vi "sub_joystick-data-conv.vi"(11 "joystick info-in":T1) -> (2 "cmd":u32, 3 "opval":cluster{dbl, dbl} {"?" format="%-1.1f"; "?" format="%-1.1f"})   [LabVIEW 2021]
uses:
  Ctrl/cmd_common.ctl
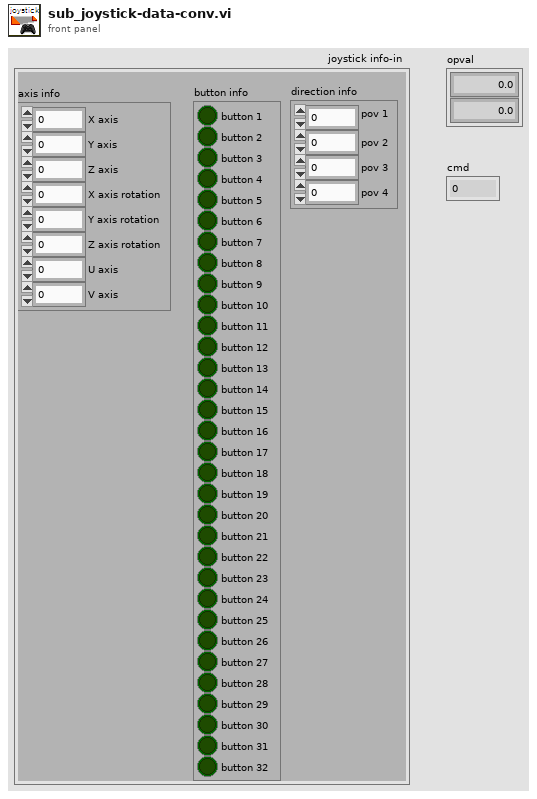
[diagram p1: front panel]
types:
  T1 = cluster{"axis info":cluster{"X axis":i32, "Y axis":i32, "Z axis":i32, "X axis rotation":i32, "Y axis rotation":i32, "Z axis rotation":i32, "U axis":i32, "V axis":i32}, "button info":cluster{"button 1":bool, "button 2":bool, "button 3":bool, "button 4":bool, "button 5":bool, "button 6":bool, "button 7":bool, "button 8":bool, "button 9":bool, "button 10":bool, "button 11":bool, "button 12":bool, "button 13":bool, "button 14":bool, "button 15":bool, "button 16":bool, "button 17":bool, "button 18":bool, "button 19":bool, "button 20":bool, "button 21":bool, "button 22":bool, "button 23":bool, "button 24":bool, "button 25":bool, "button 26":bool, "button 27":bool, "button 28":bool, "button 29":bool, "button 30":bool, "button 31":bool, "button 32":bool}, "direction info":cluster{"pov 1":i32, "pov 2":i32, "pov 3":i32, "pov 4":i32}}
  T2 = typedef "system_hw.ctl" = cluster{"UGV":enum16{"none", "Scout", "RLCar", "ASV", "Bunker"}, "Lidar 1":enum16{"none", "VLP16", "TIM571", "RPLidar A2", "RPLidar A3", "Ouster"}, "Lidar 2":enum16{"none", "VLP16", "TIM571", "RPLidar A2", "RPLidar A3"}, "GPS":enum16{"none", "NMEA 232", "Custom", "tbd"}, "Camera 1":enum16{"none", "C920", "C922", "GT1290C", "MS LifeCam"}, "Joystick":enum16{"none", "joystick"}, "sound":enum16{"none", "speaker"}, "IMU":enum16{"none", "MW-AHRSv1", "VN-100", "MTi-630", "Ellipse-D", "WT901CTTL"}, "Led":enum16{"none", "LedMatrix 8x32"}, "Camera 2":enum16{"none", "C920", "C922", "GT1290C", "MS LifeCam"}, "Camera 3":enum16{"none", "C920", "C922", "GT1290C", "MS LifeCam"}, "Camera 4":enum16{"none", "C920", "C922", "GT1290C", "MS LifeCam"}}
  T3 = enum16{"none", "Scout", "RLCar", "ASV", "Bunker"}
  T4 = typedef "cmd_common.ctl" = enum16{"read", "write"}
  T5 = typedef "joystick cfg.ctl" = cluster{"steer limit":cluster{"scale":dbl, "offset":dbl}, "speed limit":cluster{"min":dbl, "max":dbl}, "Axis":cluster{"man":dbl, "auto":dbl, "angular":T6, "linear":T6, "linear inv":bool, "ang inv":bool}}
  T6 = typedef "joy-axis.ctl" = enum16{"X axis", "Y axis", "Z axis", "X rotation", "Y rotation", "Z rotation", "U axis", "V axis"}
  T7 = cluster{"X axis":i32, "Y axis":i32, "Z axis":i32, "X axis rotation":i32, "Y axis rotation":i32, "Z axis rotation":i32, "U axis":i32, "V axis":i32}
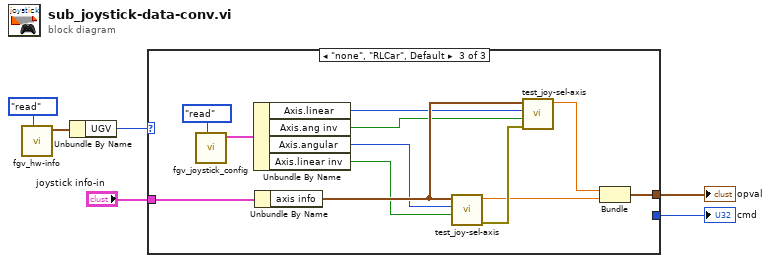
[diagram p0: block diagram]
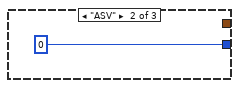
[diagram p3: hidden frame]
diagram:
  n1 = call "fgv_hw-info.vi"("cmd"=enum16{"write", "read"}."read") -> ("HW info out"=w1:T2)  [unwired: 10 in]
  n2 = Unbundle By Name(w1) -> ("UGV"=w3:T3)
  n3 = case shown="\"none\", \"RLCar\", Default" w3 {
    tunnel: [_ _ w10] -> w6
    tunnel: "joystick info-in" -> [_ _ w15]
    tunnel: [_ u32 0 _] -> w4
    frame "Scout" {
    }
    frame "ASV" {
    }
    frame "none", "RLCar", Default {
      n4 = call "fgv_joystick_config.vi"("cmd"=cmd_common."read") -> ("Joystick cfg 3"=w18:T5)  [unwired: 9 in, 1 out]
      n5 = Unbundle By Name(w18) -> ("Axis.linear"=w12:T6, "Axis.ang inv"=w11:bool, "Axis.angular"=w13:T6, "Axis.linear inv"=w14:bool)
      n6 = Unbundle By Name(w15) -> ("axis info"=w17:T7)
      n7 = call "test_joy-sel-axis.vi"("invert"=w14, "select axis"=w13, "axis info"=w17) -> ("error out"=w16:errorcluster, "x"=w8:dbl)  [unwired: 7 in]
      n8 = call "test_joy-sel-axis.vi"("error in"=w16, "invert"=w11, "select axis"=w12, "axis info"=w17) -> ("x"=w9:dbl)  [unwired: 6 in, 1 out]
      n9 = Bundle("x"=w9, "x"=w8) -> (w10:cluster{"x":dbl, "x":dbl})  [unwired: 1 in]
    }
  }
  "opval" <- w6
  "cmd" <- w4
